vi "Get_X2,Y2_from_(X,Y,dX,dY).vi"(2 "dY":dbl, 3 "dX":dbl, 4 "Y1":dbl, 5 "X1":dbl) -> (0 "Y2 = (Y1+dY)":dbl, 1 "X2 = (X1+dX)":dbl)   [LabVIEW 2013]
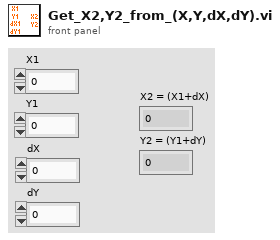
[diagram p1: front panel]
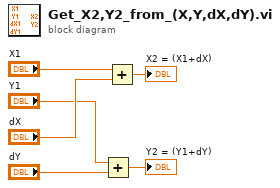
[diagram p0: block diagram]
diagram:
  n1 = Add(x="Y1", y="dY") -> (x+y=→"Y2 = (Y1+dY)":dbl)
  n2 = Add(x="X1", y="dX") -> (x+y=→"X2 = (X1+dX)":dbl)
